vi "SW_Fire_TTL_during_calibration.vi"(8 "error in (no error)":errorcluster, 9 "VISA resource in":refnum<visa-resource-name>="Tracker", 10 "Port to fire":u16(ring)=8 items=["Out 1"=1, "Out 2"=2, "Out 3"=4, "Out 4"=8], 11 "TTL pulse length, s":dbl=250.0 format="%#_13g") -> (0 "error out":errorcluster, 1 "VISA resource out":refnum<visa-resource-name>="Tracker", 3 "Time spent to process command, s":dbl)   [LabVIEW 2018, in "Tracker.lvlib"]
doc: "Fires TTL High to the TTL2 output for ~250 ms (default)."
uses:
  Tracker.lvlib
  <vilib>/Instr/_visa.llb/VISA Flush IO Buffer Mask.ctl
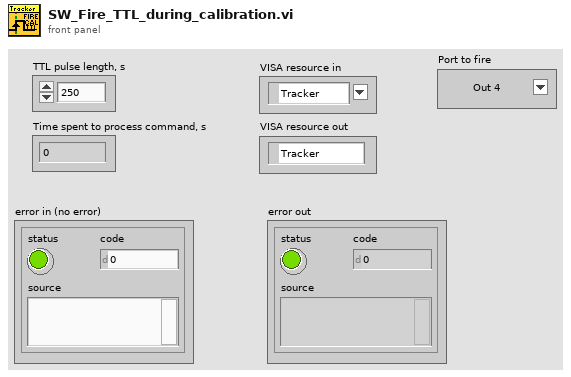
[diagram p1: front panel]
types:
  T1 = typedef "VISA Flush IO Buffer Mask.ctl" = u16
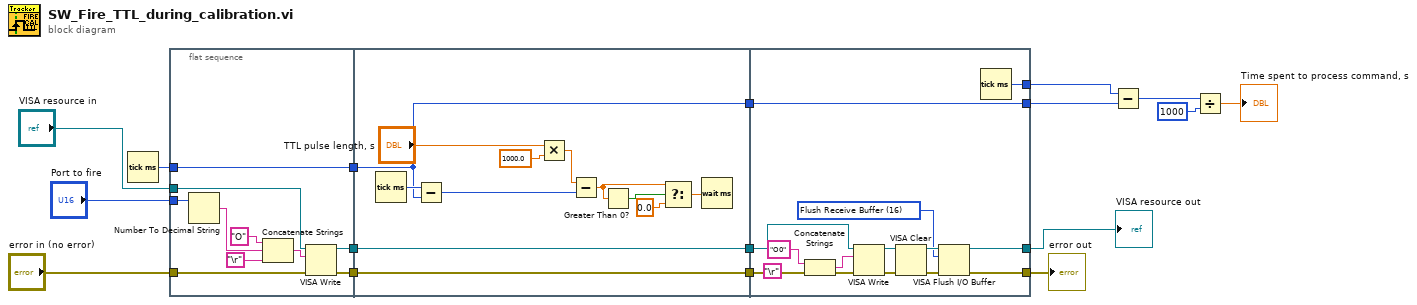
[diagram p0: block diagram]
diagram:
  n1 = Tick Count (ms)() -> (millisecond timer value=w6:u32)
  n2 = flat-sequence {
    tunnel: "VISA resource in" -> [w25]
    tunnel: [w27] -> w12
    tunnel: [w26] -> w11
    tunnel: [w24] -> w10
    tunnel: w6 -> [w24]
    tunnel: "error in (no error)" -> [w23]
    tunnel: "Port to fire" -> [w20]
    tunnel: [w39] -> w7
    tunnel: w12 -> [w39]
    tunnel: [w38] -> w8
    tunnel: w11 -> [w38]
    tunnel: w10 -> [w30]
    tunnel: [w30] -> w9
    tunnel: [w43] -> w14
    tunnel: [w44] -> w16
    tunnel: [w52] -> w4
    tunnel: [w53] -> w5
    tunnel: w9 -> [w52]
    tunnel: w8 -> [w48]
    tunnel: w7 -> [w47]
    frame #0 {
      n3 = Number To Decimal String(number=w20) -> (decimal integer string=w22:string)  [unwired: 1 in]
      n4 = Concatenate Strings("O" ("string"), w22, "\r") -> (w19:string)
      n5 = VISA Write(VISA resource name=w25, write buffer=w19, error in (no error)=w23) -> (VISA resource name out=w27:refnum<visa-resource-name>, error out=w26:errorcluster)  [unwired: 1 out]
    }
    frame #1 {
      n6 = Tick Count (ms)() -> (millisecond timer value=w37:u32)
      n7 = Subtract(x=w37, y=w30) -> (x-y=w35:u32)
      n8 = Multiply(x="TTL pulse length, s", y=1000.0) -> (x*y=w29:dbl)
      n9 = Subtract(x=w29, y=w35) -> (x-y=w32:dbl)
      n10 = Greater Than 0?(x=w32) -> (x > 0?=w34:bool)
      n11 = Select(t=w32, s=w34, f=0.0) -> (s? t:f=w33:dbl)
      n12 = Wait (ms)(milliseconds to wait=w33) -> ()  [unwired: 1 out]
    }
    frame #2 {
      w49 = T1 16 items=["Flush Receive Buffer"=16, "Write Transmit Buffer to Device"=32, "Flush Receive Buffer (No I/O)"=64, "Flush Transmit Buffer"=128] ("Mask")
      n13 = Concatenate Strings("O0" ("write buffer"), "\r") -> (w40:string)
      n14 = VISA Write(VISA resource name=w47, write buffer=w40, error in (no error)=w48) -> (VISA resource name out=w46:refnum<visa-resource-name>, error out=w45:errorcluster)  [unwired: 1 out]
      n15 = VISA Clear(VISA resource name=w46, error in (no error)=w45) -> (VISA resource name out=w50:refnum<visa-resource-name>, error out=w51:errorcluster)
      n16 = VISA Flush I/O Buffer(VISA resource name=w50, mask (16)=w49, error in (no error)=w51) -> (VISA resource name out=w44:refnum<visa-resource-name>, error out=w43:errorcluster)
      n17 = Tick Count (ms)() -> (millisecond timer value=w53:u32)
    }
  }
  n18 = Subtract(x=w5, y=w4) -> (x-y=w17:u32)
  n19 = Divide(x=w17, y=u32 1000) -> (x/y=→"Time spent to process command, s":dbl)
  "VISA resource out" <- w16
  "error out" <- w14
